vi "Cleanup client and server backup.vi"(8 "error in":errorcluster, 11 "proto File Path":path) -> (0 "error out":errorcluster)   [LabVIEW 2021, in "Script gRPC.lvlib"]
uses:
  Script gRPC.lvlib
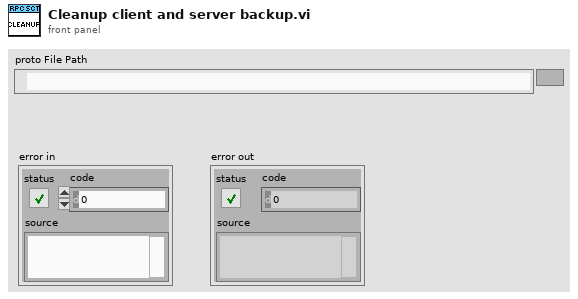
[diagram p1: front panel]
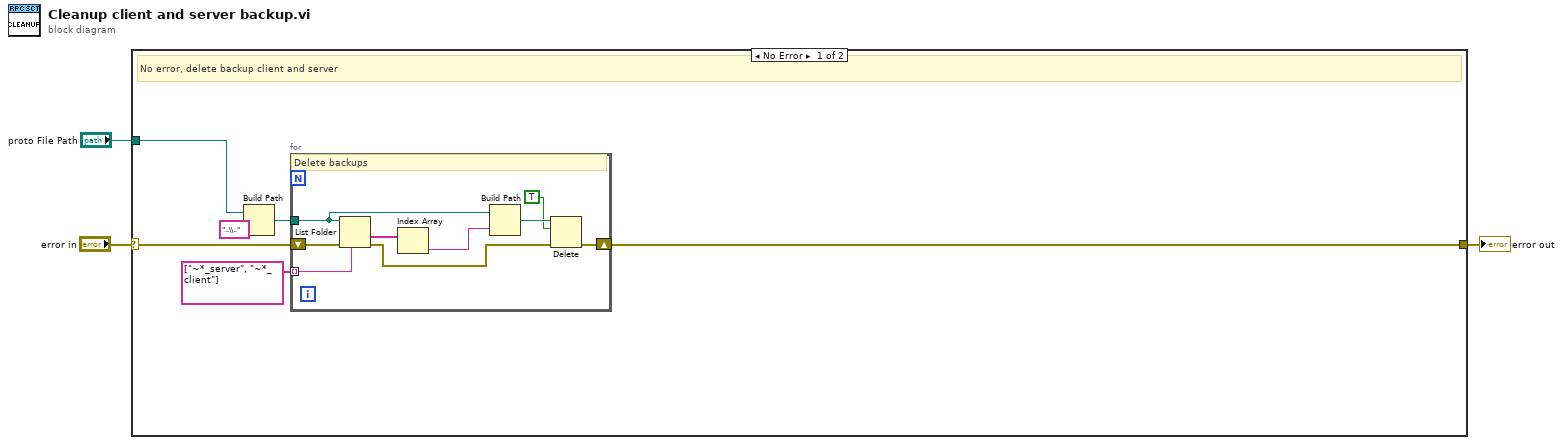
[diagram p0: block diagram]
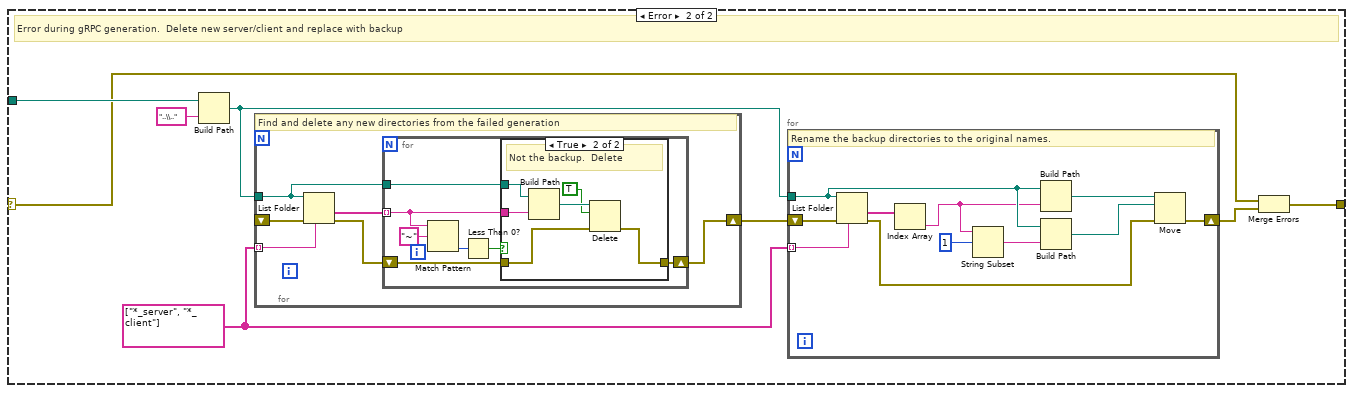
[diagram p2: hidden frame]
diagram:
  n1 = case shown="No Error" "error in" {
    selector: "error in" -> [w4 w22]
    tunnel: [w6 w21] -> w3
    tunnel: "proto File Path" -> [w5 w25]
    frame No Error {
      # "No error, delete backup client and server"
      n2 = Build Path(base path=w5, name or relative path="..\\.." ("String")) -> (appended path=w8:path)
      n3 = for {
        tunnel: w8 -> [w15]
        tunnel: string[] ["~*_server", "~*_client"] -> [w17] mode=indexing
        shift-right: [w11] -> w6
        shift-left: w4 -> [w16]
        # "Delete backups"
        n4 = List Folder(path=w15, pattern=w17, error in=w16) -> (folder names=w18:string[], error out=w12:errorcluster)  [unwired: 1 in, 2 out]
        n5 = Index Array(array=w18) -> (element=w14:string)  [unwired: 1 in]
        n6 = Build Path(base path=w15, name or relative path=w14) -> (appended path=w13:path)
        n7 = Delete(path (use dialog)=w13, entire hierarchy (F)=TRUE, error in=w12) -> (error out=w11:errorcluster)  [unwired: 2 in, 2 out]
      }
    }
    frame Error {
      w23 = string[] ["*_server", "*_client"]
      # "Error during gRPC generation.  Delete new server/client and replace with backup"
      n8 = Build Path(base path=w25, name or relative path="..\\.." ("String")) -> (appended path=w19:path)
      n9 = for {
        tunnel: w19 -> [w41]
        tunnel: w23 -> [w43] mode=indexing
        shift-right: [w39] -> w24
        shift-left: _ -> [w42]
        # "Find and delete any new directories from the failed generation"
        n10 = List Folder(path=w41, pattern=w43, error in=w42) -> (folder names=w38:string[], error out=w40:errorcluster)  [unwired: 1 in, 2 out]
        n11 = for {
          tunnel: w41 -> [w50]
          shift-right: [w48] -> w39
          shift-left: w40 -> [w49]
          tunnel: w38 -> [w44] mode=indexing
          n12 = Match Pattern(string=w44, regular expression="~") -> (offset past match=w46:i32)  [unwired: 1 in, 3 out]
          n13 = Less Than 0?(x=w46) -> (x < 0?=w45:bool)
          n14 = case shown="True" w45 {
            tunnel: w50 -> [_ w57]
            tunnel: w49 -> [w51 w55]
            tunnel: [w51 w54] -> w48
            tunnel: w44 -> [_ w53]
            frame False {
              # "Backup.  Do nothing"
            }
            frame True {
              # "Not the backup.  Delete"
              n15 = Build Path(base path=w57, name or relative path=w53) -> (appended path=w56:path)
              n16 = Delete(path (use dialog)=w56, entire hierarchy (F)=TRUE, error in=w55) -> (error out=w54:errorcluster)  [unwired: 2 in, 2 out]
            }
          }
        }
      }
      n17 = for {
        tunnel: w19 -> [w35]
        tunnel: w23 -> [w32] mode=indexing
        shift-right: [w30] -> w20
        shift-left: w24 -> [w31]
        # "Rename the backup directories to the original names."
        n18 = List Folder(path=w35, pattern=w32, error in=w31) -> (folder names=w37:string[], error out=w33:errorcluster)  [unwired: 1 in, 2 out]
        n19 = Index Array(array=w37) -> (element=w29:string)  [unwired: 1 in]
        n20 = String Subset(string=w29, offset (0)=1) -> (substring=w28:string)  [unwired: 1 in]
        n21 = Build Path(base path=w35, name or relative path=w29) -> (appended path=w36:path)
        n22 = Build Path(base path=w35, name or relative path=w28) -> (appended path=w34:path)
        n23 = Move(source path=w36, error in=w33, 10:w34) -> (error out=w30:errorcluster)  [unwired: 2 in, 2 out]
      }
      n24 = Merge Errors(w22, w20) -> (w21:errorcluster)
    }
  }
  "error out" <- w3
